vi "DDS Write Register.vi"(6 "channel number (1)":u8=1 min=1 max=4 step=1, 7 "# RAM words (0)":i32, 8 "error in (no error)":errorcluster, 9 "Write Data":u8[](array[numeric]), 10 "Register":T3, 11 "DDS ref in":T1={"NI USB-8451 device reference"="", "DIO port"=0, "Serial Clock Rate [kHz]"=1000}) -> (0 "error out":errorcluster, 2 "Read data":u8[](array[numeric]), 3 "DDS ref out":T1={"NI USB-8451 device reference"="", "DIO port"=0, "Serial Clock Rate [kHz]"=1000})   [LabVIEW 2013, in "DDS.lvlib"]
doc: "Writes data to the specified register in the specified channel. The number of bytes written must equal the register size."
uses:
  DDS.lvlib
  Controls/AD9910 registers.ctl
  Controls/DDS Box Device Reference.ctl
  <vilib>/ni845x/ni845x.llb/ni845xControl.ctl
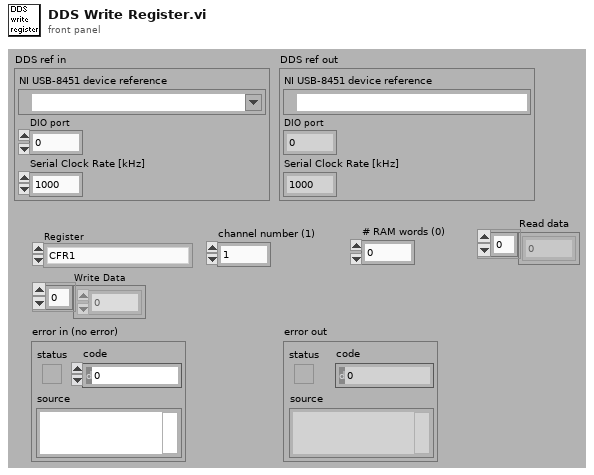
[diagram p1: front panel]
types:
  T1 = typedef "DDS.lvlib/DDS Box Device Reference.ctl" = cluster{"NI USB-8451 device reference":T2, "DIO port":u8, "Serial Clock Rate [kHz]":u16}
  T2 = typedef "ni845xControl.ctl" = refnum<k21>
  T3 = typedef "DDS.lvlib/AD9910 registers.ctl" = enum16{"CFR1", "CFR2", "CFR3", "Auxiliary DAC Control", "I/0 Update Rate", "Frequency Tuning Word", "Phase Offset Word", "Amplitude Scale Factor", "Multichip Sync", "Digital Ramp Limit", "Digital Ramp Step Size", "Digital Ramp Rate", "Single Tone Profile 0", "Single Tone Profile 1", "Single Tone Profile 2", "Single Tone Profile 3", "Single Tone Profile 4", "Single Tone Profile 5", "Single Tone Profile 6", "Single Tone Profile 7", "RAM Profile 0", "RAM Profile 1", "RAM Profile 2", "RAM Profile 3", "RAM Profile 4", "RAM Profile 5", "RAM Profile 6", "RAM Profile 7", "RAM"}
  T4 = typedef "ni845xSpiScriptControl.ctl" = refnum<k20>
  T5 = typedef "DDS.lvlib/DDS CS pins.ctl" = enum8{"IO reset", "Ch. 4 CS", "Ch. 3 CS", "Ch. 2 CS", "Ch. 1 CS"}
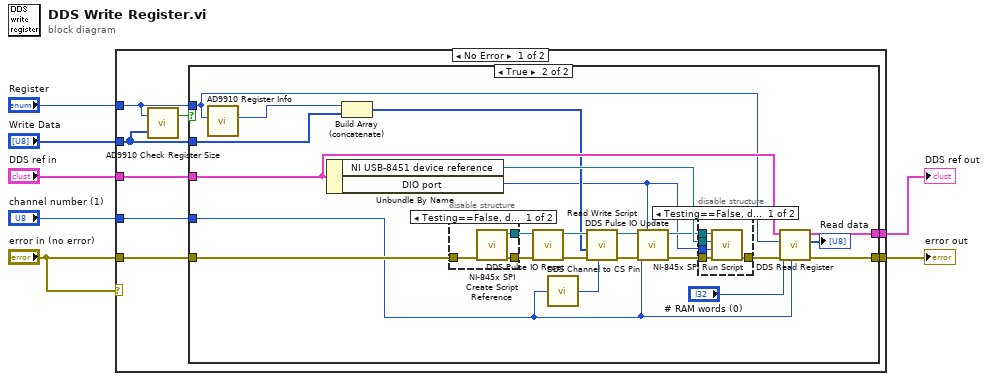
[diagram p0: block diagram]
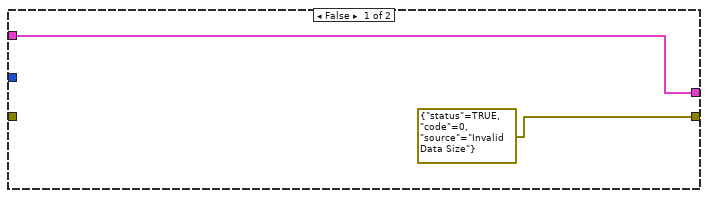
[diagram p2: hidden frame]
diagram:
  n1 = case shown="No Error" "error in (no error)" {
    tunnel: "error in (no error)" -> [w15 w52]
    tunnel: "DDS ref in" -> [w14 w51]
    tunnel: "Register" -> [w10 _]
    tunnel: [w13 w52] -> w5
    tunnel: "Write Data" -> [w11 _]
    tunnel: "channel number (1)" -> [w12 _]
    tunnel: [w8 w51] -> w1
    frame No Error {
      n2 = call "AD9910 Check Register Size.vi"("Write Data"=w11, "Register"=w10) -> ("passed"=w9:bool)  [unwired: 1 out]
      n3 = case shown="True" w9 {
        tunnel: w15 -> [_ w40]
        tunnel: w14 -> [w16 w39]
        tunnel: w10 -> [_ w35]
        tunnel: w11 -> [_ w38]
        tunnel: [errorcluster {"status"=TRUE, "code"=0, "source"="Invalid Data Size"} ("error in (no error)") w36] -> w13
        tunnel: w12 -> [_ w18]
        tunnel: [w16 w34] -> w8
        frame False {
        }
        frame True {
          n4 = call "AD9910 Register Info.vi"("Register"=w35) -> ("Address"=w37:u8)  [unwired: 9 in, 1 out]
          n5 = Unbundle By Name(w39) -> ("NI USB-8451 device reference"=w29:T2, "DIO port"=w22:u8)
          n6 = Build Array (concatenate)(w37, w38) -> (w28:u8[])
          n7 = disable-structure shown="Testing==False, default" {
            disable-tunnel: w40 -> [w49 w50]
            disable-tunnel: [w48 _] -> w33
            disable-tunnel: [w47 w50] -> w32
            frame condition #0 (active) {
              n8 = call <vilib>:"NI-845x SPI Create Script Reference.vi"("error in (no error)"=w49) -> ("error out"=w47:errorcluster, "spi script reference"=w48:T4)  [unwired: 9 in]
            }
            frame condition #1 {
            }
          }
          n9 = call "DDS Pulse IO Reset.vi"("error in (no error)"=w32, "spi script reference in"=w33) -> ("error out"=w31:errorcluster, "spi script reference out"=w30:T4)  [unwired: 8 in]
          n10 = call "DDS Channel to CS Pin.vi"("channel number (1)"=w18) -> ("CS pin"=w23:T5)
          n11 = call "Read Write Script.vi"("chip select (0)"=w23, "error in (no error)"=w31, "Write Data"=w28, "spi script reference in"=w30) -> ("error out"=w27:errorcluster, "spi script reference out"=w26:T4)  [unwired: 5 in, 1 out]
          n12 = call "DDS Pulse IO Update.vi"("port number (0)"=w22, "error in (no error)"=w27, "channel number (1)"=w18, "spi script reference in"=w26) -> ("error out"=w24:errorcluster, "spi script reference out"=w25:T4)  [unwired: 6 in]
          n13 = disable-structure shown="Testing==False, default" {
            disable-tunnel: w29 -> [w45 _]
            disable-tunnel: [w44 w46] -> w21
            disable-tunnel: w25 -> [w43 _]
            disable-tunnel: w24 -> [w42 w46]
            disable-tunnel: w22 -> [w41 _]
            frame condition #0 (active) {
              n14 = call <vilib>:"NI-845x SPI Run Script.vi"("error in (no error)"=w42, "port (0)"=w41, "device reference in"=w45, "spi script reference in"=w43) -> ("error out"=w44:errorcluster)  [unwired: 5 in, 2 out]
            }
            frame condition #1 {
            }
          }
          n15 = call "DDS Read Register.vi"("channel number (1)"=w18, "error in (no error)"=w21, "# RAM words (0)"="# RAM words (0)", "Register"=w35, "DDS ref in"=w39) -> ("error out"=w36:errorcluster, "Read data"=→"Read data":u8[], "DDS ref out"=w34:T1)  [unwired: 4 in]
        }
      }
    }
    frame Error {
    }
  }
  "error out" <- w5
  "DDS ref out" <- w1
